vi "Global_Serial.vi"() -> ()   [LabVIEW 2015]
panel:
  out "VISA resource name":refnum<visa-resource-name>
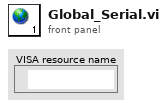
[diagram p1: front panel]
diagram:
